vi "AlliGator Convert Phasor to Phasor Plot Point.vi"(9 "Phasor Plot Reference Points":T3, 11 "Phasor":T1) -> (3 "Phasor Plot Point":T2)   [LabVIEW 2021, in "AlliGator Phasor Plot.lvlib"]
doc: "Converts phasor value to Phasor Plot image coordinates."
uses:
  AlliGator Phasor Plot Reference Points.ctl
  Phasor/Phasor (g, s).ctl
  d67848f9-f11e-415d-897b-94393b5bed14.vi
  AlliGator Phasor Plot.lvlib
  AlliGator Phasor Ratio.lvlib
  Phasor/Phasor.lvlib
panel:
  # "see the AlliGator License on the block diagram (Ctrl+E or Window:Show Block Diagram)"
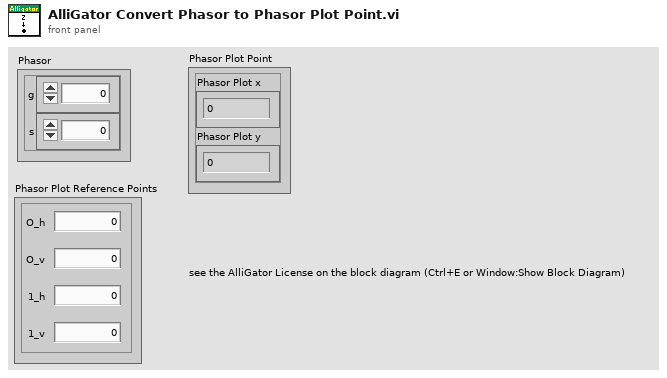
[diagram p1: front panel]
types:
  T1 = typedef "Phasor.lvlib/Phasor (g, s).ctl" = cluster{"g":dbl, "s":dbl}
  T2 = cluster{"Phasor Plot x":dbl, "Phasor Plot y":dbl}
  T3 = typedef "AlliGator Phasor Ratio.lvlib/AlliGator Phasor Plot Reference Points.ctl" = cluster{"O_h":dbl, "O_v":dbl, "1_h":dbl, "1_v":dbl}
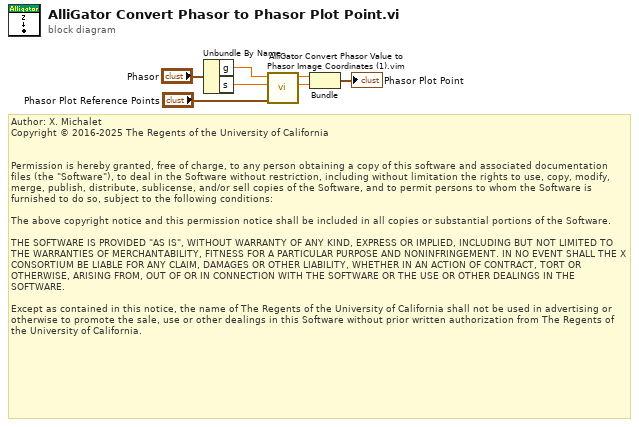
[diagram p0: block diagram]
diagram:
  # "Author: X. Michalet\nCopyright © 2016-2025 The Regents of the University of California\n \n\nPermission is hereby granted, free of charge, to any person obtaining a copy of this software and associated documentation files (the \"Software\"), to deal in the Software without restriction, including without limitation the rights to use, copy, modify, merge, publish, distribute, sublicense, and/or sell copies of the Software, and to permit persons to whom the Software is furnished to do so, subject to the following conditions:\n\nThe above copyright notice and this permission notice shall be included in all copies or substantial portions of the Software.\n\nTHE SOFTWARE IS PROVIDED \"AS IS\", WITHOUT WARRANTY OF ANY KIND, EXPRESS OR IMPLIED, INCLUDING BUT NOT LIMITED TO THE WARRANTIES OF MERCHANTABILITY, FITNESS FOR A PARTICULAR PURPOSE AND NONINFRINGEMENT. IN NO EVENT SHALL THE X CONSORTIUM BE LIABLE FOR ANY CLAIM, DAMAGES OR OTHER LIABILITY, WHETHER IN AN ACTION OF CONTRACT, TORT OR OTHERWISE, ARISING FROM, OUT OF OR IN CONNECTION WITH THE SOFTWARE OR THE USE OR OTHER DEALINGS IN THE SOFTWARE.\n\nExcept as contained in this notice, the name of The Regents of the University of California shall not be used in advertising or otherwise to promote the sale, use or other dealings in this Software without prior written authorization from The Regents of the University of California."
  n1 = Unbundle By Name("Phasor") -> ("g"=w2:dbl, "s"=w3:dbl)
  n2 = call "AlliGator Convert Phasor Value to Phasor Image Coordinates (1).vim"("Phasor Plot Reference Points"="Phasor Plot Reference Points", "Phasor s"=w3, "Phasor g"=w2) -> ("Phasor Plot y"=w5:dbl, "Phasor Plot x"=w4:dbl)  [unwired: 7 in]
  n3 = Bundle("Phasor Plot x"=w4, "Phasor Plot y"=w5) -> (→"Phasor Plot Point":T2)  [unwired: 1 in]
